vi "Targeting Unit.vi"(0 "Main Interface":T6, 1 "Focus and Tracking":T3, 2 "Guided Approach":T4, 3 "Controls":T1, 4 "Start Coordinates [pix]":refnum<vi>, 5 "Manipulator Interface":T10, 7 "Target":T9, 9 "Tip":T8, 11 "Error In":errorcluster, 12 "System of Reference Interface":T7, 13 "Calibration":T5, 14 "State":refnum<vi>) -> (15 "Error Out":errorcluster)   [LabVIEW 2012, in "Targeting Unit.lvlib"]
uses:
  Targeting Unit.lvlib
  <vilib>/Analysis/Matrix/Datatypes/RealMatrix.ctl
  State.ctl
  <vilib>/Analysis/Matrix/NI_Matrix.lvlib
panel:
  out "Final Reference [um]":T2
  out "Initial Reference [um]":T2
  out "Exit":bool
  out "XmF":dbl format="%.2f"
  out "XmI":dbl format="%.2f"
  out "Final [pix]":cluster{"X":sgl, "Y":sgl}
  out "Initial [pix]":cluster{"X":sgl, "Y":sgl}
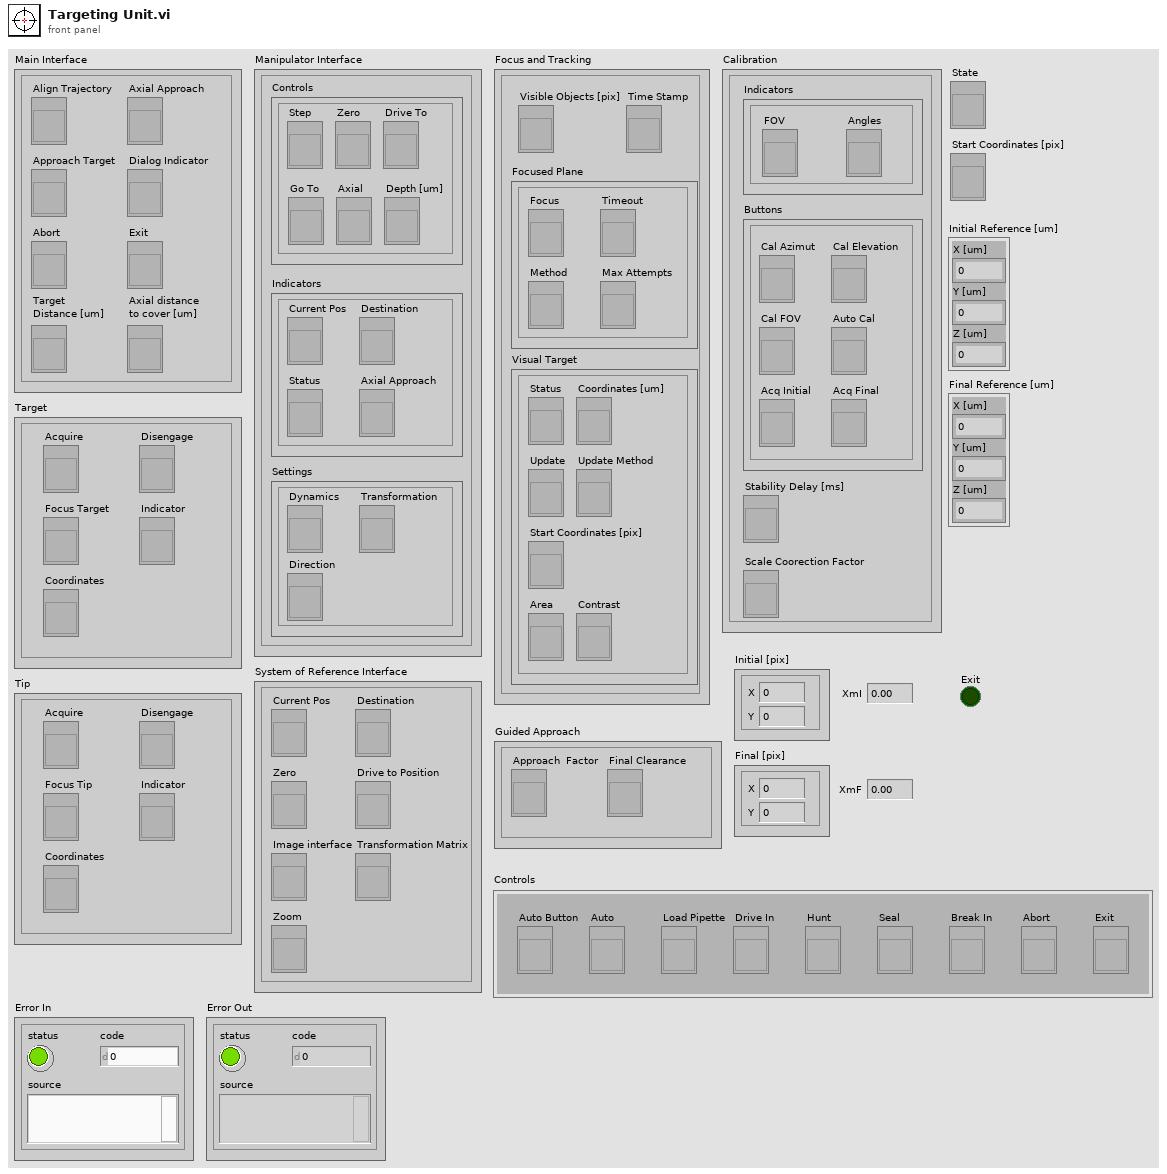
[diagram p1: front panel]
types:
  T1 = cluster{"Load Pipette":refnum<vi>, "Drive In":refnum<vi>, "Hunt":refnum<vi>, "Seal":refnum<vi>, "Break In":refnum<vi>, "Abort":refnum<vi>, "Exit":refnum<vi>, "Auto":refnum<vi>, "Auto Button":refnum<vi>}
  T2 = cluster{"X [um]":dbl, "Y [um]":dbl, "Z [um]":dbl}
  T3 = cluster{"Focused Plane":cluster{"Focus":refnum<vi>, "Timeout":refnum<vi>, "Max Attempts":refnum<vi>, "Method":refnum<vi>}, "Time Stamp":refnum<vi>, "Visual Target":cluster{"Coordinates [um]":refnum<vi>, "Status":refnum<vi>, "Update":refnum<vi>, "Update Method":refnum<vi>, "Start Coordinates [pix]":refnum<vi>, "Area":refnum<vi>, "Contrast":refnum<vi>}, "Visible Objects [pix]":refnum<vi>}
  T4 = cluster{"Approach  Factor":refnum<vi>, "Final Clearance":refnum<vi>}
  T5 = cluster{"Indicators":cluster{"FOV":refnum<vi>, "Angles":refnum<vi>}, "Buttons":cluster{"Cal FOV":refnum<vi>, "Cal Azimut":refnum<vi>, "Cal Elevation":refnum<vi>, "Auto Cal":refnum<vi>, "Acq Initial":refnum<vi>, "Acq Final":refnum<vi>}, "Stability Delay [ms]":refnum<vi>, "Scale Coorection Factor":refnum<vi>}
  T6 = cluster{"Exit":refnum<vi>, "Abort":refnum<vi>, "Align Trajectory":refnum<vi>, "Axial Approach":refnum<vi>, "Dialog Indicator":refnum<vi>, "Approach Target":refnum<vi>, "Target\nDistance [um]":refnum<vi>, "Axial distance\nto cover [um]":refnum<vi>}
  T7 = cluster{"Current Pos":refnum<vi>, "Image interface":refnum<vi>, "Transformation Matrix":refnum<vi>, "Zero":refnum<vi>, "Destination":refnum<vi>, "Drive to Position":refnum<vi>, "Zoom":refnum<vi>}
  T8 = cluster{"Coordinates":refnum<vi>, "Acquire":refnum<vi>, "Disengage":refnum<vi>, "Indicator":refnum<vi>, "Focus Tip":refnum<vi>}
  T9 = cluster{"Coordinates":refnum<vi>, "Acquire":refnum<vi>, "Disengage":refnum<vi>, "Indicator":refnum<vi>, "Focus Target":refnum<vi>}
  T10 = cluster{"Indicators":cluster{"Current Pos":refnum<vi>, "Destination":refnum<vi>, "Status":refnum<vi>, "Axial Approach":refnum<vi>}, "Settings":cluster{"Dynamics":refnum<vi>, "Transformation":refnum<vi>, "Direction":refnum<vi>}, "Controls":cluster{"Zero":refnum<vi>, "Step":refnum<vi>, "Drive To":refnum<vi>, "Go To":refnum<vi>, "Axial":refnum<vi>, "Depth [um]":refnum<vi>}}
  T11 = typedef "NI_Matrix.lvlib/RealMatrix.ctl" = dbl[][]
  T12 = cluster{"X [um]":bool, "Y [um]":bool, "Z [um]":bool}
  T13 = cluster{"Global Rectangle":i32[], "Contours":cluster{"Contour Type":u32, "ROI Type":u32, "Points":i32[]}[]}
  T14 = typedef "IMAQ Point" = cluster{"X":sgl, "Y":sgl}
  T15 = typedef "State.ctl" = enum16{"READY", "LOAD", "LOCALIZATION", "HUNTING", "SEAL", "BREAKIN", "WCR", "ALIGN", "APPROACH", "TARGETING"}
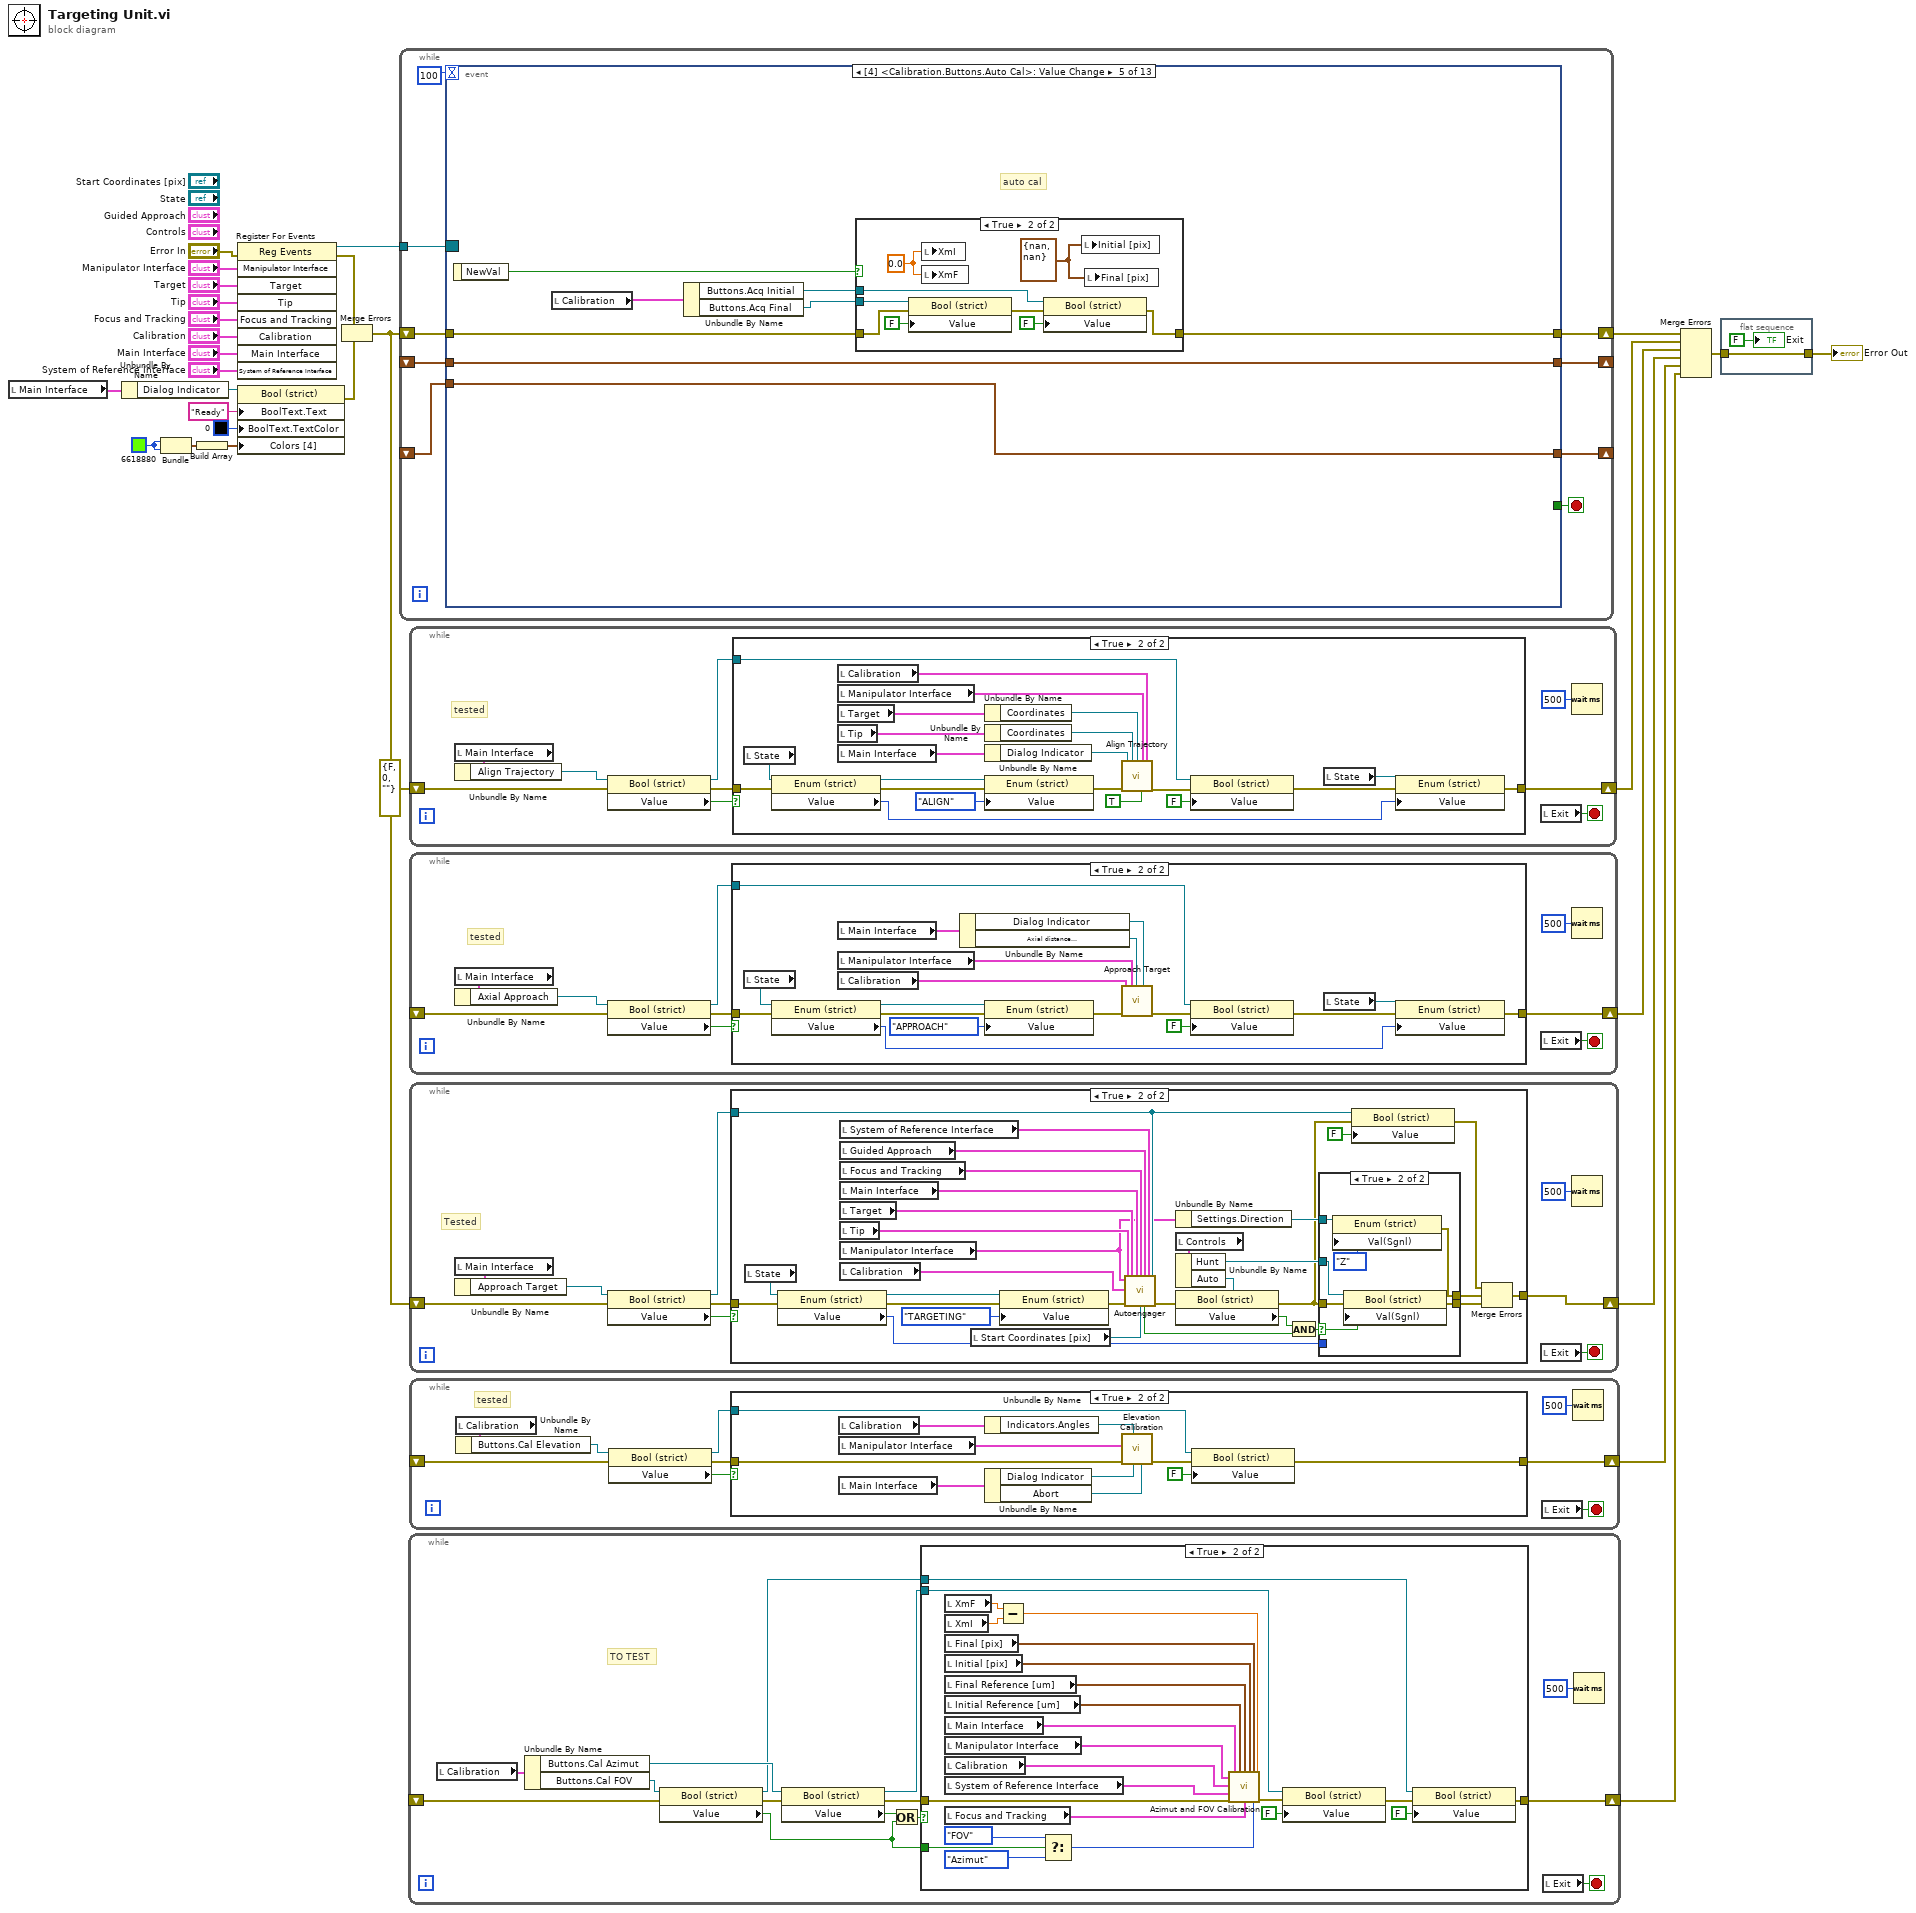
[diagram p0: block diagram]
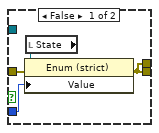
[diagram p3: hidden frame]
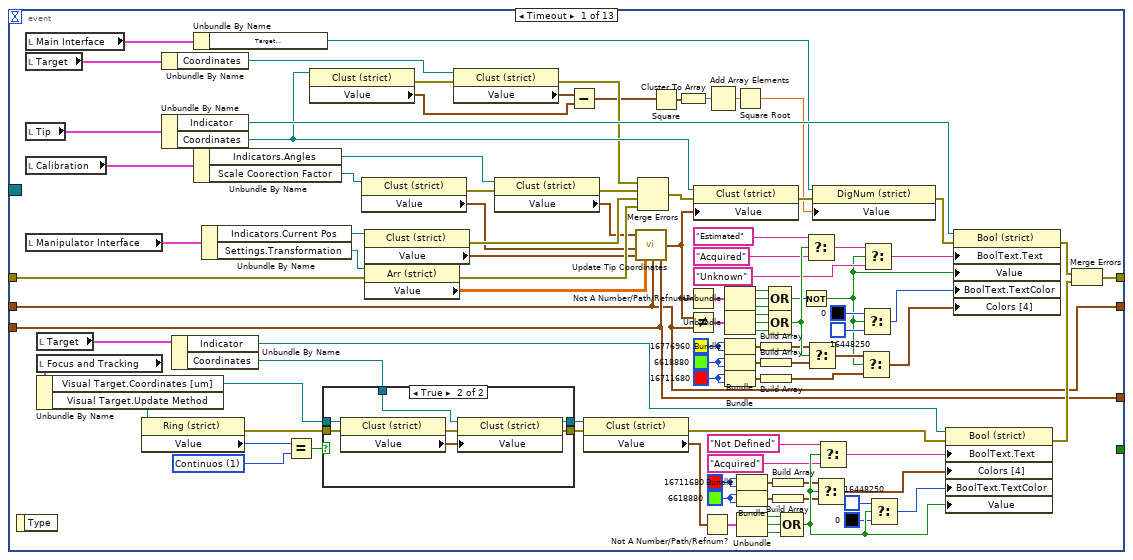
[diagram p8: hidden frame]
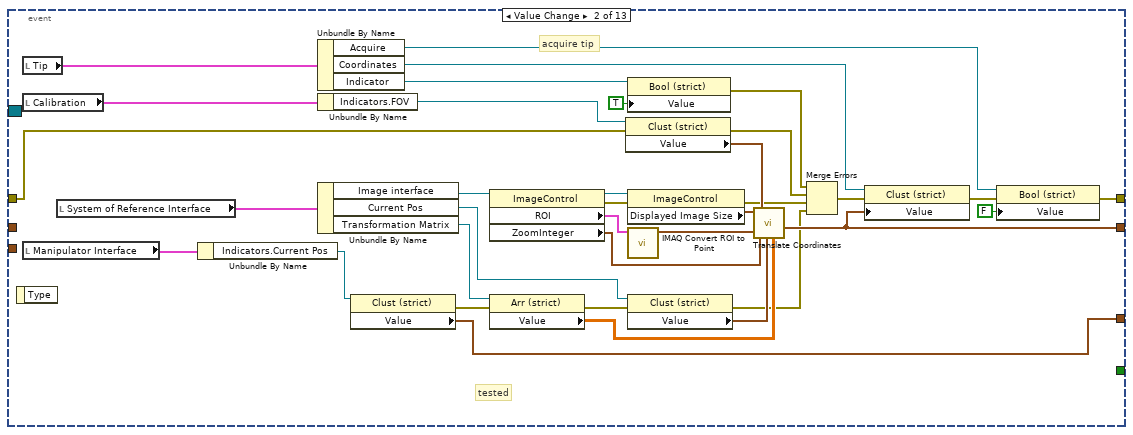
[diagram p10: hidden frame]
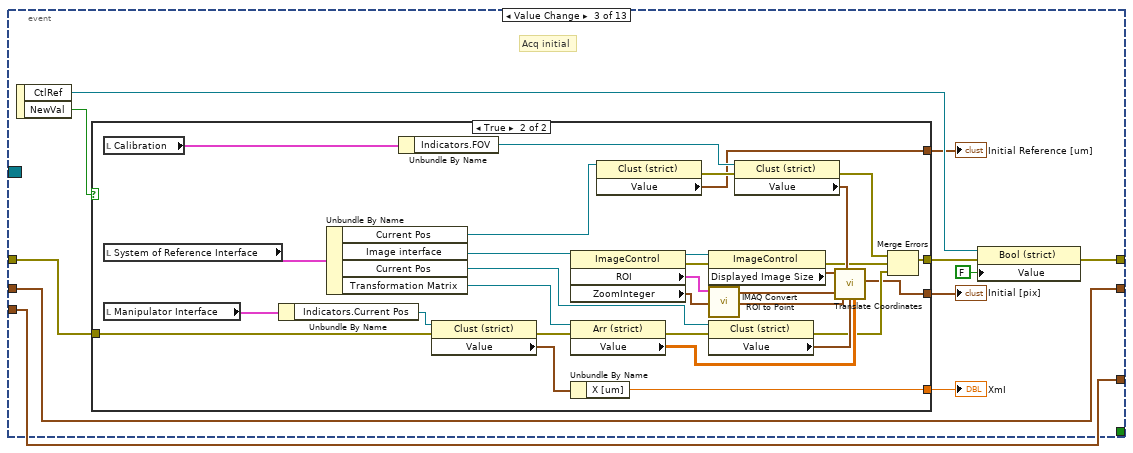
[diagram p11: hidden frame]
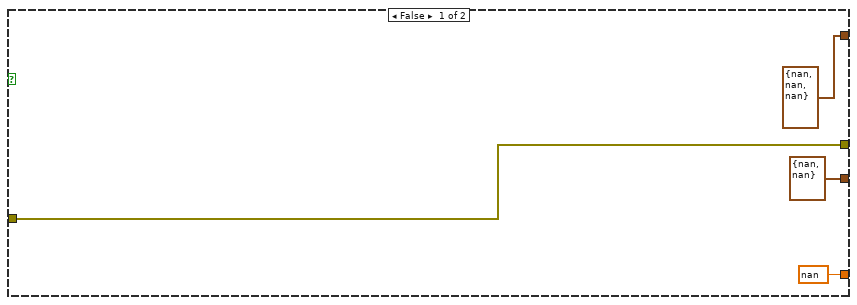
[diagram p12: hidden frame]
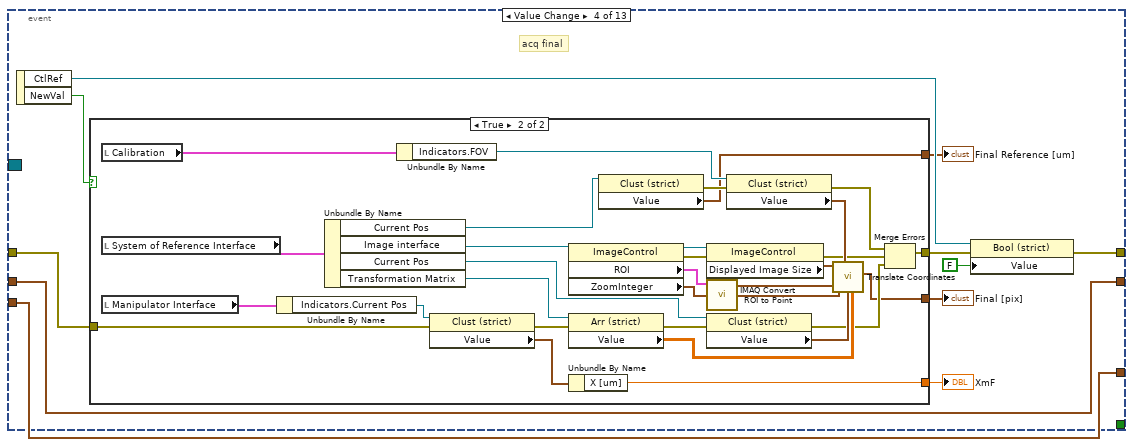
[diagram p13: hidden frame]
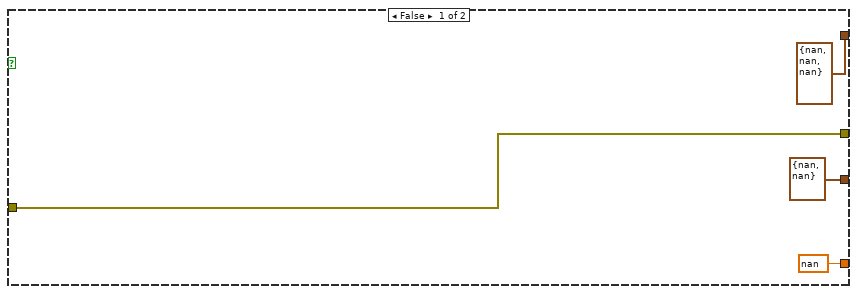
[diagram p14: hidden frame]
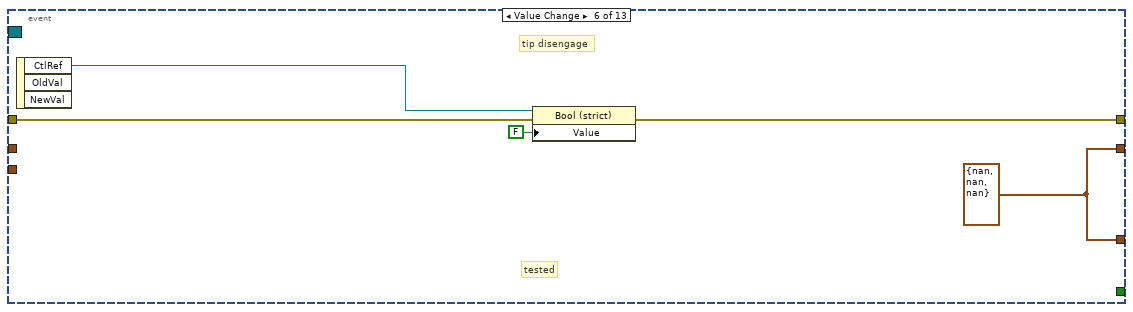
[diagram p16: hidden frame]
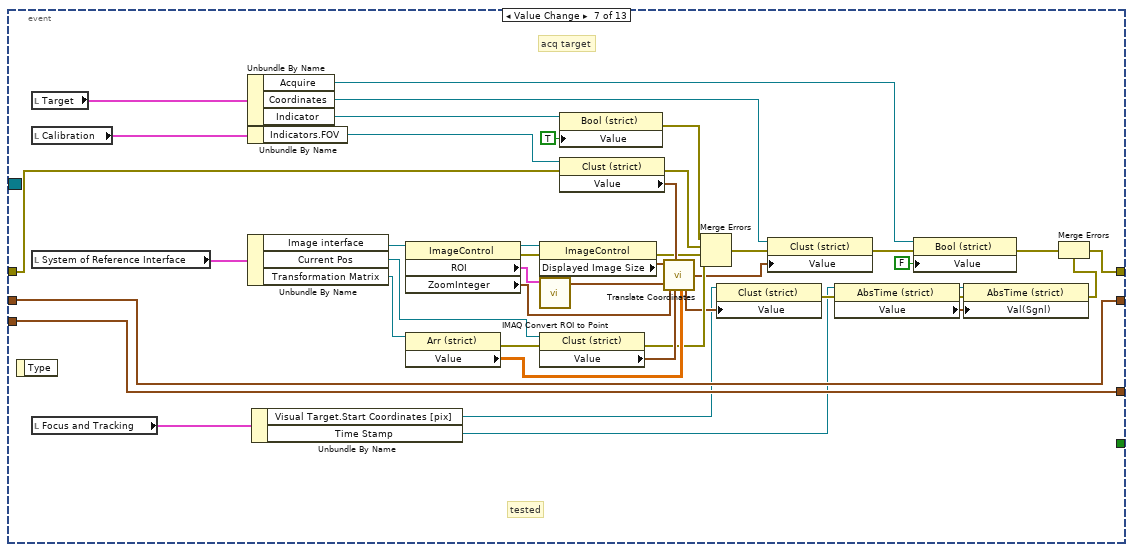
[diagram p17: hidden frame]
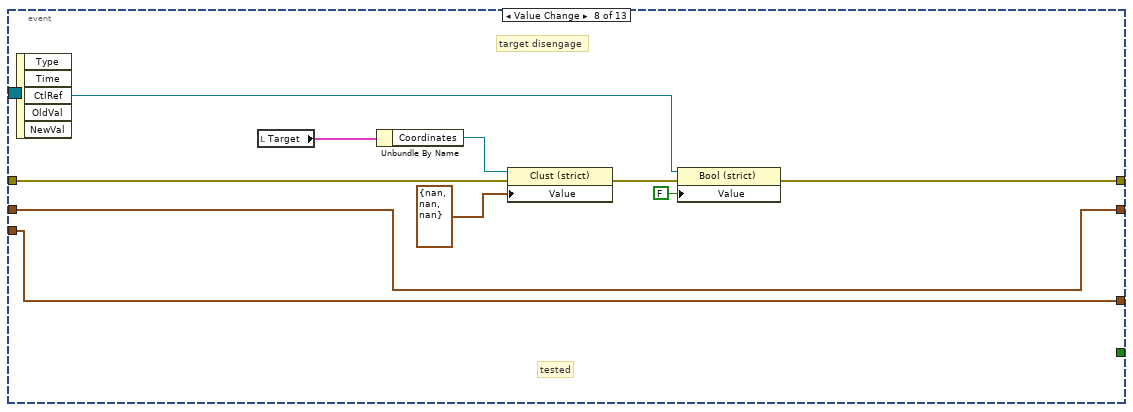
[diagram p18: hidden frame]
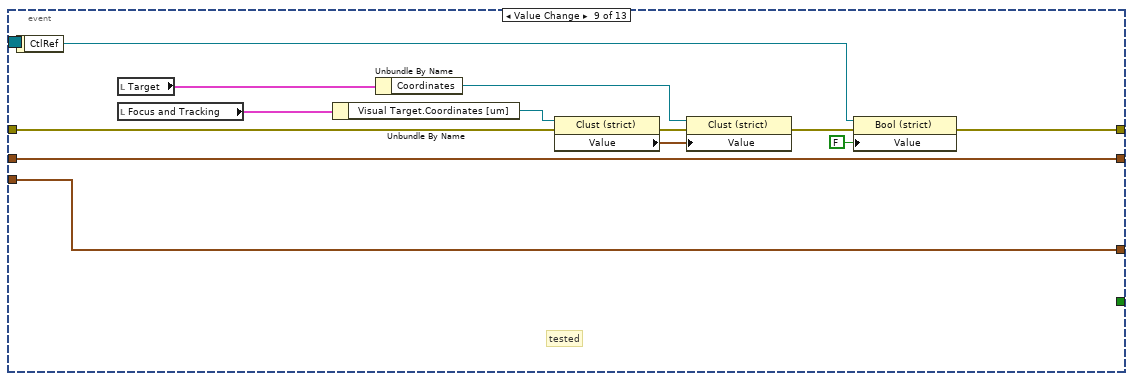
[diagram p19: hidden frame]
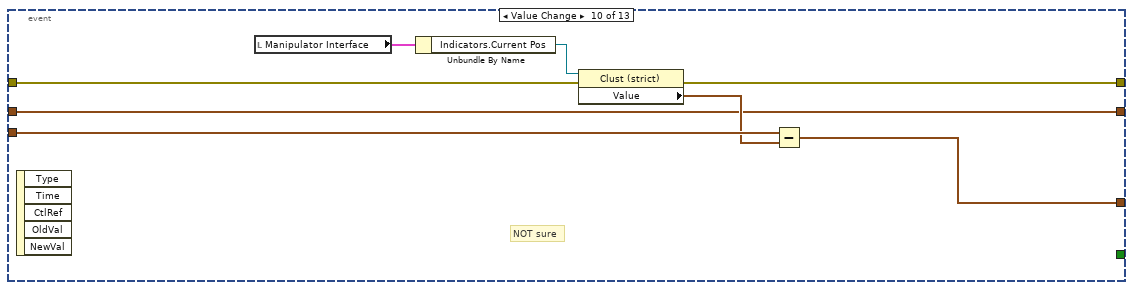
[diagram p20: hidden frame]
diagram:
  w8 = u32 6618880
  n1 = local read "Main Interface"() -> (w3:T6)
  n2 = Unbundle By Name(w3) -> ("Dialog Indicator"=w2:refnum<vi>)
  n3 = Bundle(w8, w8) -> (w7:cluster{u32, u32})  [unwired: 1 in]
  n4 = Build Array(w7) -> (w4:cluster{u32, u32}[])
  n5 = register-events(error in="Error In", "Manipulator Interface", "Target", "Tip", "Focus and Tracking", "Calibration", "Main Interface", "System of Reference Interface") -> (reference out=w23:refnum<event-registration>, error out=w18:errorcluster)  [unwired: 1 in]
  n6 = property class="Bool (strict)"(reference=w2, "BoolText.Text"="Ready" ("Boolean Text.Text"), "BoolText.TextColor"=u32 0, "Colors [4]"=w4) -> (error out=w6:errorcluster)  [unwired: 1 in, 1 out]
  n7 = Merge Errors(w18, w6) -> (w10:errorcluster)
  n8 = while {
    tunnel: w23 -> [w37]
    shift-right: [w35] -> _
    shift-left: _ -> [w34]
    shift-right: [w36] -> _
    shift-left: _ -> [w33]
    shift-right: [w32] -> w17
    shift-left: w10 -> [w29]
    stop <- w30 stop-if-true
    n9 = event shown="[4] <Calibration.Buttons.Auto Cal>: Value Change" {
      selector: w37 -> [_ _ _ _ _ _ _ _ _ _ _ _ _]
      dyn-events: _ -> [_ _ _ _ _ _ _ _ _ _ _ _ _]
      timeout: 100 -> [_ _ _ _ _ _ _ _ _ _ _ _ _]
      tunnel: [w57 w176 w186 w239 w280 w296 w313 w341 w355 w363 w374 w405 w422] -> w36
      tunnel: [w59 w150 w185 w237 w279 w296 w312 w342 w354 w370 w372 w404 w423] -> w35
      tunnel: w34 -> [w59 _ w185 w237 w279 _ w312 w342 w354 w369 w372 w404 w423]
      tunnel: w33 -> [w57 _ w186 w239 w280 _ w313 w341 w355 w363 w373 w405 w422]
      tunnel: [w73 w158 w190 w233 w276 w293 w301 w348 w352 w365 w379 w391 w425] -> w32
      tunnel: w29 -> [w87 w149 w192 w238 w277 w294 w297 w345 w356 w366 w383 w398 w425]
      tunnel: [_ _ _ _ _ _ _ _ _ _ _ _ w424] -> w30
      event Timeout {
        w63 = 1 items=["On Demand", "Continuos"] ("Target Update Method")
        w120 = u32 16711680
        w110 = u32 6618880
        w107 = u32 16776960
        w95 = u32 6618880
        w92 = u32 16711680
        n10 = event-data() -> ()  [unwired: 1 in, 1 out]
        n11 = local read "Main Interface"() -> (w38:T6)
        n12 = local read "Target"() -> (w47:T9)
        n13 = local read "Tip"() -> (w134:T8)
        n14 = local read "Calibration"() -> (w135:T5)
        n15 = local read "Manipulator Interface"() -> (w137:T10)
        n16 = local read "Target"() -> (w80:T9)
        n17 = local read "Focus and Tracking"() -> (w65:T3)
        n18 = Unbundle By Name(w65) -> ("Visual Target.Coordinates [um]"=w58:refnum<vi>, "Visual Target.Update Method"=w64:refnum<vi>)
        n19 = property class="Ring (strict)"(reference=w64) -> (error out=w61:errorcluster, "Value"=w62:i32)  [unwired: 1 in, 1 out]
        n20 = Unbundle By Name(w47) -> ("Coordinates"=w46:refnum<vi>)
        n21 = Unbundle By Name(w134) -> ("Indicator"=w72:refnum<vi>, "Coordinates"=w50:refnum<vi>)
        n22 = Unbundle By Name(w80) -> ("Indicator"=w69:refnum<vi>, "Coordinates"=w67:refnum<vi>)
        n23 = Unbundle By Name(w38) -> ("Target\nDistance [um]"=w44:refnum<vi>)
        n24 = Unbundle By Name(w135) -> ("Indicators.Angles"=w136:refnum<vi>, "Scale Coorection Factor"=w55:refnum<vi>)
        n25 = Unbundle By Name(w137) -> ("Indicators.Current Pos"=w139:refnum<vi>, "Settings.Transformation"=w138:refnum<vi>)
        n26 = Equal?(x=w62, y=w63) -> (x = y?=w60:bool)
        n27 = property class="Clust (strict)"(reference=w50) -> (error out=w45:errorcluster, "Value"=w42:T2)  [unwired: 1 in, 1 out]
        n28 = case shown="True" w60 {
          tunnel: [w141 w148] -> w68
          tunnel: w67 -> [w140 w146]
          tunnel: [w140 w147] -> w66
          tunnel: w58 -> [_ w145]
          tunnel: w61 -> [w141 w144]
          frame False {
          }
          frame True {
            n29 = property class="Clust (strict)"(reference=w145, error in=w144) -> (error out=w142:errorcluster, "Value"=w143:cluster{"X":dbl, "Y":dbl, "Z":dbl})  [unwired: 1 out]
            n30 = property class="Clust (strict)"(reference=w146, error in=w142, "Value"=w143) -> (reference out=w147:refnum<vi>, error out=w148:errorcluster)
          }
        }
        n31 = property class="Clust (strict)"(reference=w55) -> (error out=w56:errorcluster, "Value"=w54:cluster{"Kx":dbl, "Ky":dbl, "Kz":dbl})  [unwired: 1 in, 1 out]
        n32 = property class="Clust (strict)"(reference=w139) -> (error out=w85:errorcluster, "Value"=w82:T2)  [unwired: 1 in, 1 out]
        n33 = property class="Arr (strict)"(reference=w138, error in=w87) -> (error out=w84:errorcluster, "Value"=w133:T11)  [unwired: 1 out]
        n34 = property class="Clust (strict)"(reference=w46, error in=w45) -> (error out=w41:errorcluster, "Value"=w43:T2)  [unwired: 1 out]
        n35 = property class="Clust (strict)"(reference=w136, error in=w56) -> (error out=w86:errorcluster, "Value"=w83:cluster{"Azimut":dbl, "Elevation":dbl})  [unwired: 1 out]
        n36 = Subtract(x=w43, y=w42) -> (x-y=w40:T2)
        n37 = property class="Clust (strict)"(reference=w66, error in=w68) -> (error out=w70:errorcluster, "Value"=w101:T2)  [unwired: 1 out]
        n38 = call "Update Tip Coordinates.vi"("Scale Coorection Factor"=w54, "Angles"=w83, "Transformation Matrix"=w133, "Initial Manipulator Coordinates"=w59, "Initial Tip Coordinates"=w57, "Current Manipulator Coordinates"=w82) -> ("Current Coordinates"=w79:T2)  [unwired: 5 in]
        n39 = Merge Errors(w41, w86, w85, w84) -> (w81:errorcluster)
        n40 = Square(x=w40) -> (x^2=w51:T2)
        n41 = Cluster To Array(cluster=w51) -> (array=w52:dbl[])
        n42 = Not A Number/Path/Refnum?(number/path/refnum=w79) -> (NaN/Path/Refnum?=w115:T12)
        n43 = Not Equal?(x=w79, y=w57) -> (x != y?=w88:T12)
        n44 = property class="Clust (strict)"(reference=w50, error in=w81, "Value"=w79) -> (error out=w49:errorcluster)  [unwired: 1 out]
        n45 = Not A Number/Path/Refnum?(number/path/refnum=w101) -> (NaN/Path/Refnum?=w102:T12)
        n46 = Add Array Elements(numeric array=w52) -> (sum=w53:dbl)
        n47 = Unbundle(w115) -> ("X [um]"=w116:bool, "Y [um]"=w117:bool, "Z [um]"=w118:bool)
        n48 = Unbundle(w88) -> ("X [um]"=w89:bool, "Y [um]"=w90:bool, "Z [um]"=w91:bool)
        n49 = Bundle(w107, w107) -> (w108:cluster{u32, u32})  [unwired: 1 in]
        n50 = Bundle(w110, w110) -> (w111:cluster{u32, u32})  [unwired: 1 in]
        n51 = Bundle(w120, w120) -> (w121:cluster{u32, u32})  [unwired: 1 in]
        n52 = Square Root(x=w53) -> (sqrt(x)=w39:dbl)
        n53 = Bundle(w92, w92) -> (w93:cluster{u32, u32})  [unwired: 1 in]
        n54 = Bundle(w95, w95) -> (w96:cluster{u32, u32})  [unwired: 1 in]
        n55 = Unbundle(w102) -> ("X [um]"=w103:bool, "Y [um]"=w104:bool, "Z [um]"=w105:bool)
        n56 = Build Array(w108) -> (w109:cluster{u32, u32}[])
        n57 = Build Array(w111) -> (w112:cluster{u32, u32}[])
        n58 = Build Array(w121) -> (w124:cluster{u32, u32}[])
        n59 = Compound Arithmetic op=OR(w116, w117, w118) -> (w119:bool)
        n60 = Compound Arithmetic op=OR(w89, w90, w91) -> (w126:bool)
        n61 = Build Array(w93) -> (w94:cluster{u32, u32}[])
        n62 = Build Array(w96) -> (w97:cluster{u32, u32}[])
        n63 = Compound Arithmetic op=OR(w103, w104, w105) -> (w132:bool)
        n64 = Not(x=w119) -> (.not. x?=w77:bool)
        n65 = Select(t="Estimated" ("Boolean Text.Text"), s=w126, f="Acquired" ("Boolean Text.Text")) -> (s? t:f=w122:string)
        n66 = Select(t=w109, s=w126, f=w112) -> (s? t:f=w125:cluster{u32, u32}[])
        n67 = property class="DigNum (strict)"(reference=w44, error in=w49, "Value"=w39) -> (error out=w48:errorcluster)  [unwired: 1 out]
        n68 = Select(t=w94, s=w132, f=w97) -> (s? t:f=w100:cluster{u32, u32}[])
        n69 = Select(t="Not Defined" ("Boolean Text.Text"), s=w132, f="Acquired" ("Boolean Text.Text")) -> (s? t:f=w106:string)
        n70 = Select(t=w125, s=w77, f=w124) -> (s? t:f=w75:cluster{u32, u32}[])
        n71 = Select(t=u32 0, s=w77, f=u32 16448250) -> (s? t:f=w76:u32)
        n72 = Select(t=w122, s=w77, f="Unknown" ("Boolean Text.Text")) -> (s? t:f=w78:string)
        n73 = Select(t=u32 16448250, s=w132, f=u32 0) -> (s? t:f=w131:u32)
        n74 = property class="Bool (strict)"(reference=w69, error in=w70, "BoolText.Text"=w106, "Colors [4]"=w100, "BoolText.TextColor"=w131, "Value"=w132) -> (error out=w71:errorcluster)  [unwired: 1 out]
        n75 = property class="Bool (strict)"(reference=w72, error in=w48, "BoolText.Text"=w78, "Value"=w77, "BoolText.TextColor"=w76, "Colors [4]"=w75) -> (error out=w74:errorcluster)  [unwired: 1 out]
        n76 = Merge Errors(w74, w71) -> (w73:errorcluster)
      }
      event Value Change {
        # "acquire tip"
        # "tested"
        n77 = event-data() -> ()  [unwired: 1 in, 1 out]
        n78 = local read "Tip"() -> (w177:T8)
        n79 = local read "Calibration"() -> (w179:T5)
        n80 = local read "Manipulator Interface"() -> (w175:T10)
        n81 = local read "System of Reference Interface"() -> (w163:T7)
        n82 = Unbundle By Name(w175) -> ("Indicators.Current Pos"=w174:refnum<vi>)
        n83 = Unbundle By Name(w177) -> ("Acquire"=w173:refnum<vi>, "Coordinates"=w154:refnum<vi>, "Indicator"=w153:refnum<vi>)
        n84 = Unbundle By Name(w179) -> ("Indicators.FOV"=w178:refnum<vi>)
        n85 = Unbundle By Name(w163) -> ("Image interface"=w167:refnum<vi>, "Current Pos"=w157:refnum<vi>, "Transformation Matrix"=w172:refnum<vi>)
        n86 = property class="Clust (strict)"(reference=w174) -> (error out=w156:errorcluster, "Value"=w150:T2)  [unwired: 1 in, 1 out]
        n87 = property on="Property Node" class="ImageControl"(reference=w167) -> (reference out=w168:refnum<vi>, error out=w166:errorcluster, "ROI"=w180:T13, "ZoomInteger"=w151:cluster{"X":i32, "Y":i32})  [unwired: 1 in]
        n88 = property class="Arr (strict)"(reference=w172, error in=w156) -> (error out=w164:errorcluster, "Value"=w182:T11)  [unwired: 1 out]
        n89 = property class="Clust (strict)"(reference=w178, error in=w149) -> (error out=w162:errorcluster, "Value"=w171:cluster{"FOVx [um]":dbl, "FOVy [um]":dbl})  [unwired: 1 out]
        n90 = property class="Bool (strict)"(reference=w153, "Value"=TRUE) -> (error out=w152:errorcluster)  [unwired: 1 in, 1 out]
        n91 = property class="ImageControl"(reference=w168, error in=w166) -> (error out=w161:errorcluster, "Displayed Image Size"=w169:cluster{"Width":u32, "Height":u32})  [unwired: 1 out]
        n92 = call "IMAQ Convert ROI to Point"("ROI Descriptor"=w180) -> ("Point"=w170:T14)  [unwired: 1 in, 8 out]
        n93 = property class="Clust (strict)"(reference=w157, error in=w164) -> (error out=w159:errorcluster, "Value"=w165:T2)  [unwired: 1 out]
        n94 = call "Translate Coordinates.vi"("Transformation Matrix"=w182, "Coordinates [pix]"=w170, "FOV"=w171, "Visualiser Zoom"=w151, "Scope Position"=w165, "Image Area"=w169) -> ("Target Coordinates"=w176:T2)  [unwired: 4 in, 1 out]
        n95 = Merge Errors(w152, w162, w161, w159) -> (w160:errorcluster)
        n96 = property class="Clust (strict)"(reference=w154, error in=w160, "Value"=w176) -> (error out=w155:errorcluster)  [unwired: 1 out]
        n97 = property class="Bool (strict)"(reference=w173, error in=w155, "Value"=FALSE) -> (error out=w158:errorcluster)  [unwired: 1 out]
      }
      event Value Change {
        # "Acq initial"
        n98 = event-data() -> ("CtlRef"=w188:refnum<vi>, "NewVal"=w191:bool)  [unwired: 1 in]
        n99 = case shown="True" w191 {
          tunnel: [w198 w207] -> w189
          tunnel: [cluster{"X":sgl, "Y":sgl} {"X"=nan, "Y"=nan} ("coordinates [pix]") w203] -> w194
          tunnel: [nan ("X [um]") w205] -> w193
          tunnel: w192 -> [w198 w204]
          tunnel: [T2 {"X [um]"=nan, "Y [um]"=nan, "Z [um]"=nan} ("Value") w200] -> w184
          frame False {
          }
          frame True {
            n100 = local read "Calibration"() -> (w226:T5)
            n101 = local read "System of Reference Interface"() -> (w213:T7)
            n102 = local read "Manipulator Interface"() -> (w224:T10)
            n103 = Unbundle By Name(w224) -> ("Indicators.Current Pos"=w223:refnum<vi>)
            n104 = Unbundle By Name(w213) -> ("Current Pos"=w202:refnum<vi>, "Image interface"=w217:refnum<vi>, "Current Pos"=w209:refnum<vi>, "Transformation Matrix"=w222:refnum<vi>)
            n105 = Unbundle By Name(w226) -> ("Indicators.FOV"=w225:refnum<vi>)
            n106 = property class="Clust (strict)"(reference=w223, error in=w204) -> (error out=w208:errorcluster, "Value"=w206:T2)  [unwired: 1 out]
            n107 = property on="Property Node" class="ImageControl"(reference=w217) -> (reference out=w218:refnum<vi>, error out=w216:errorcluster, "ROI"=w227:T13, "ZoomInteger"=w199:cluster{"X":i32, "Y":i32})  [unwired: 1 in]
            n108 = property class="Arr (strict)"(reference=w222, error in=w208) -> (error out=w214:errorcluster, "Value"=w228:T11)  [unwired: 1 out]
            n109 = Unbundle By Name(w206) -> ("X [um]"=w205:dbl)
            n110 = property class="Clust (strict)"(reference=w202) -> (error out=w201:errorcluster, "Value"=w200:T2)  [unwired: 1 in, 1 out]
            n111 = property class="ImageControl"(reference=w218, error in=w216) -> (error out=w211:errorcluster, "Displayed Image Size"=w219:cluster{"Width":u32, "Height":u32})  [unwired: 1 out]
            n112 = call "IMAQ Convert ROI to Point"("ROI Descriptor"=w227) -> ("Point"=w220:T14)  [unwired: 1 in, 8 out]
            n113 = property class="Clust (strict)"(reference=w209, error in=w214) -> (error out=w210:errorcluster, "Value"=w215:T2)  [unwired: 1 out]
            n114 = property class="Clust (strict)"(reference=w225, error in=w201) -> (error out=w212:errorcluster, "Value"=w221:cluster{"FOVx [um]":dbl, "FOVy [um]":dbl})  [unwired: 1 out]
            n115 = call "Translate Coordinates.vi"("Transformation Matrix"=w228, "Coordinates [pix]"=w220, "FOV"=w221, "Visualiser Zoom"=w199, "Scope Position"=w215, "Image Area"=w219) -> ("coordinates [pix]"=w203:cluster{"X":sgl, "Y":sgl})  [unwired: 4 in, 1 out]
            n116 = Merge Errors(w212, w211, w210) -> (w207:errorcluster)
          }
        }
        "Initial [pix]" <- w194
        "XmI" <- w193
        "Initial Reference [um]" <- w184
        n117 = property class="Bool (strict)"(reference=w188, error in=w189, "Value"=FALSE) -> (error out=w190:errorcluster)  [unwired: 1 out]
      }
      event Value Change {
        # "acq final"
        n118 = event-data() -> ("CtlRef"=w230:refnum<vi>, "NewVal"=w231:bool)  [unwired: 1 in]
        n119 = case shown="True" w231 {
          tunnel: [w243 w252] -> w232
          tunnel: [cluster{"X":sgl, "Y":sgl} {"X"=nan, "Y"=nan} ("coordinates [pix]") w251] -> w236
          tunnel: [nan ("X [um]") w249] -> w235
          tunnel: w238 -> [w243 w248]
          tunnel: [T2 {"X [um]"=nan, "Y [um]"=nan, "Z [um]"=nan} ("Value") w245] -> w229
          frame False {
          }
          frame True {
            n120 = local read "Calibration"() -> (w271:T5)
            n121 = local read "System of Reference Interface"() -> (w258:T7)
            n122 = local read "Manipulator Interface"() -> (w269:T10)
            n123 = Unbundle By Name(w269) -> ("Indicators.Current Pos"=w268:refnum<vi>)
            n124 = Unbundle By Name(w258) -> ("Current Pos"=w246:refnum<vi>, "Image interface"=w262:refnum<vi>, "Current Pos"=w254:refnum<vi>, "Transformation Matrix"=w267:refnum<vi>)
            n125 = Unbundle By Name(w271) -> ("Indicators.FOV"=w270:refnum<vi>)
            n126 = property class="Clust (strict)"(reference=w268, error in=w248) -> (error out=w253:errorcluster, "Value"=w250:T2)  [unwired: 1 out]
            n127 = property on="Property Node" class="ImageControl"(reference=w262) -> (reference out=w263:refnum<vi>, error out=w261:errorcluster, "ROI"=w272:T13, "ZoomInteger"=w244:cluster{"X":i32, "Y":i32})  [unwired: 1 in]
            n128 = property class="Arr (strict)"(reference=w267, error in=w253) -> (error out=w259:errorcluster, "Value"=w273:T11)  [unwired: 1 out]
            n129 = Unbundle By Name(w250) -> ("X [um]"=w249:dbl)
            n130 = property class="Clust (strict)"(reference=w246) -> (error out=w247:errorcluster, "Value"=w245:T2)  [unwired: 1 in, 1 out]
            n131 = property class="ImageControl"(reference=w263, error in=w261) -> (error out=w256:errorcluster, "Displayed Image Size"=w264:cluster{"Width":u32, "Height":u32})  [unwired: 1 out]
            n132 = call "IMAQ Convert ROI to Point"("ROI Descriptor"=w272) -> ("Point"=w265:T14)  [unwired: 1 in, 8 out]
            n133 = property class="Clust (strict)"(reference=w254, error in=w259) -> (error out=w255:errorcluster, "Value"=w260:T2)  [unwired: 1 out]
            n134 = property class="Clust (strict)"(reference=w270, error in=w247) -> (error out=w257:errorcluster, "Value"=w266:cluster{"FOVx [um]":dbl, "FOVy [um]":dbl})  [unwired: 1 out]
            n135 = call "Translate Coordinates.vi"("Transformation Matrix"=w273, "Coordinates [pix]"=w265, "FOV"=w266, "Visualiser Zoom"=w244, "Scope Position"=w260, "Image Area"=w264) -> ("coordinates [pix]"=w251:cluster{"X":sgl, "Y":sgl})  [unwired: 4 in, 1 out]
            n136 = Merge Errors(w257, w256, w255) -> (w252:errorcluster)
          }
        }
        "Final [pix]" <- w236
        "XmF" <- w235
        "Final Reference [um]" <- w229
        n137 = property class="Bool (strict)"(reference=w230, error in=w232, "Value"=FALSE) -> (error out=w233:errorcluster)  [unwired: 1 out]
      }
      event Value Change {
        # "auto cal"
        n138 = event-data() -> ("NewVal"=w281:bool)  [unwired: 1 in]
        n139 = local read "Calibration"() -> (w278:T5)
        n140 = Unbundle By Name(w278) -> ("Buttons.Acq Initial"=w274:refnum<vi>, "Buttons.Acq Final"=w275:refnum<vi>)
        n141 = case shown="True" w281 {
          tunnel: w277 -> [w282 w289]
          tunnel: [w282 w287] -> w276
          tunnel: w275 -> [_ w286]
          tunnel: w274 -> [_ w285]
          frame False {
          }
          frame True {
            w290 = 0.0 ("XmI")
            w291 = cluster{"X":sgl, "Y":sgl} {"X"=nan, "Y"=nan} ("Initial [pix]")
            n142 = property class="Bool (strict)"(reference=w286, error in=w289, "Value"=FALSE) -> (error out=w288:errorcluster)  [unwired: 1 out]
            n143 = local write "XmI"(w290) -> ()
            n144 = local write "XmF"(w290) -> ()
            n145 = property class="Bool (strict)"(reference=w285, error in=w288, "Value"=FALSE) -> (error out=w287:errorcluster)  [unwired: 1 out]
            n146 = local write "Initial [pix]"(w291) -> ()
            n147 = local write "Final [pix]"(w291) -> ()
          }
        }
      }
      event Value Change {
        w296 = T2 {"X [um]"=nan, "Y [um]"=nan, "Z [um]"=nan} ("Value")
        # "tip disengage"
        # "tested"
        n148 = event-data() -> ("CtlRef"=w292:refnum<vi>)  [unwired: 1 in, 2 out]
        n149 = property class="Bool (strict)"(reference=w292, error in=w294, "Value"=FALSE) -> (error out=w293:errorcluster)  [unwired: 1 out]
      }
      event Value Change {
        # "acq target"
        # "tested"
        n150 = event-data() -> ()  [unwired: 1 in, 1 out]
        n151 = local read "Target"() -> (w333:T9)
        n152 = local read "Calibration"() -> (w335:T5)
        n153 = local read "System of Reference Interface"() -> (w322:T7)
        n154 = local read "Focus and Tracking"() -> (w311:T3)
        n155 = Unbundle By Name(w333) -> ("Acquire"=w332:refnum<vi>, "Coordinates"=w316:refnum<vi>, "Indicator"=w315:refnum<vi>)
        n156 = Unbundle By Name(w335) -> ("Indicators.FOV"=w334:refnum<vi>)
        n157 = Unbundle By Name(w322) -> ("Image interface"=w326:refnum<vi>, "Current Pos"=w317:refnum<vi>, "Transformation Matrix"=w331:refnum<vi>)
        n158 = Unbundle By Name(w311) -> ("Visual Target.Start Coordinates [pix]"=w308:refnum<vi>, "Time Stamp"=w303:refnum<vi>)
        n159 = property on="Property Node" class="ImageControl"(reference=w326) -> (reference out=w327:refnum<vi>, error out=w325:errorcluster, "ROI"=w336:T13, "ZoomInteger"=w298:cluster{"X":i32, "Y":i32})  [unwired: 1 in]
        n160 = property class="Arr (strict)"(reference=w331) -> (error out=w323:errorcluster, "Value"=w338:T11)  [unwired: 1 in, 1 out]
        n161 = property class="ImageControl"(reference=w327, error in=w325) -> (error out=w320:errorcluster, "Displayed Image Size"=w328:cluster{"Width":u32, "Height":u32})  [unwired: 1 out]
        n162 = call "IMAQ Convert ROI to Point"("ROI Descriptor"=w336) -> ("Point"=w329:T14)  [unwired: 1 in, 8 out]
        n163 = property class="Clust (strict)"(reference=w317, error in=w323) -> (error out=w318:errorcluster, "Value"=w324:T2)  [unwired: 1 out]
        n164 = property class="Bool (strict)"(reference=w315, "Value"=TRUE) -> (error out=w314:errorcluster)  [unwired: 1 in, 1 out]
        n165 = property class="Clust (strict)"(reference=w334, error in=w297) -> (error out=w321:errorcluster, "Value"=w330:cluster{"FOVx [um]":dbl, "FOVy [um]":dbl})  [unwired: 1 out]
        n166 = call "Translate Coordinates.vi"("Transformation Matrix"=w338, "Coordinates [pix]"=w329, "FOV"=w330, "Visualiser Zoom"=w298, "Scope Position"=w324, "Image Area"=w328) -> ("Target Coordinates"=w309:T2, "coordinates [pix]"=w310:cluster{"X":sgl, "Y":sgl})  [unwired: 4 in]
        n167 = Merge Errors(w314, w321, w320, w318) -> (w319:errorcluster)
        n168 = property class="Clust (strict)"(reference=w308, "Value"=w310) -> (error out=w304:errorcluster)  [unwired: 1 in, 1 out]
        n169 = property class="Clust (strict)"(reference=w316, error in=w319, "Value"=w309) -> (error out=w302:errorcluster)  [unwired: 1 out]
        n170 = property class="AbsTime (strict)"(reference=w303, error in=w304) -> (reference out=w307:refnum<vi>, error out=w306:errorcluster, "Value"=w305:timestamp)
        n171 = property class="Bool (strict)"(reference=w332, error in=w302, "Value"=FALSE) -> (error out=w300:errorcluster)  [unwired: 1 out]
        n172 = property class="AbsTime (strict)"(reference=w307, error in=w306, "Val(Sgnl)"=w305) -> (error out=w299:errorcluster)  [unwired: 1 out]
        n173 = Merge Errors(w300, w299) -> (w301:errorcluster)
      }
      event Value Change {
        # "target disengage"
        # "tested"
        n174 = event-data() -> ("CtlRef"=w340:refnum<vi>)  [unwired: 1 in, 4 out]
        n175 = local read "Target"() -> (w344:T9)
        n176 = Unbundle By Name(w344) -> ("Coordinates"=w343:refnum<vi>)
        n177 = property class="Clust (strict)"(reference=w343, error in=w345, "Value"=T2 {"X [um]"=nan, "Y [um]"=nan, "Z [um]"=nan}) -> (error out=w346:errorcluster)  [unwired: 1 out]
        n178 = property class="Bool (strict)"(reference=w340, error in=w346, "Value"=FALSE) -> (error out=w348:errorcluster)  [unwired: 1 out]
      }
      event Value Change {
        # "tested"
        n179 = event-data() -> ("CtlRef"=w351:refnum<vi>)  [unwired: 1 in]
        n180 = local read "Target"() -> (w362:T9)
        n181 = local read "Focus and Tracking"() -> (w360:T3)
        n182 = Unbundle By Name(w360) -> ("Visual Target.Coordinates [um]"=w359:refnum<vi>)
        n183 = Unbundle By Name(w362) -> ("Coordinates"=w361:refnum<vi>)
        n184 = property class="Clust (strict)"(reference=w359, error in=w356) -> (error out=w357:errorcluster, "Value"=w358:cluster{"X":dbl, "Y":dbl, "Z":dbl})  [unwired: 1 out]
        n185 = property class="Clust (strict)"(reference=w361, error in=w357, "Value"=w358) -> (error out=w353:errorcluster)  [unwired: 1 out]
        n186 = property class="Bool (strict)"(reference=w351, error in=w353, "Value"=FALSE) -> (error out=w352:errorcluster)  [unwired: 1 out]
      }
      event Value Change {
        # "NOT sure"
        n187 = event-data() -> ()  [unwired: 1 in, 5 out]
        n188 = local read "Manipulator Interface"() -> (w367:T10)
        n189 = Unbundle By Name(w367) -> ("Indicators.Current Pos"=w368:refnum<vi>)
        n190 = property class="Clust (strict)"(reference=w368, error in=w366) -> (error out=w365:errorcluster, "Value"=w364:T2)  [unwired: 1 out]
        n191 = Subtract(x=w369, y=w364) -> (x-y=w370:T2)
      }
      event Value Change {
        # "initial manip"
        # "initial tip"
        # "Tested"
        n192 = event-data() -> ()  [unwired: 1 in, 5 out]
        n193 = local read "Target"() -> (w381:T9)
        n194 = local read "System of Reference Interface"() -> (w384:T7)
        n195 = Unbundle By Name(w381) -> ("Coordinates"=w378:refnum<vi>)
        n196 = Unbundle By Name(w384) -> ("Current Pos"=w385:refnum<vi>)
        n197 = property class="Clust (strict)"(reference=w385, error in=w383) -> (error out=w380:errorcluster, "Value"=w371:T2)  [unwired: 1 out]
        n198 = property class="Clust (strict)"(reference=w378, error in=w380) -> (reference out=w377:refnum<vi>, error out=w382:errorcluster, "Value"=w376:T2)
        n199 = Subtract(x=w376, y=w371) -> (x-y=w375:T2)
        n200 = Subtract(x=w373, y=w371) -> (x-y=w374:T2)
        n201 = property class="Clust (strict)"(reference=w377, error in=w382, "Value"=w375) -> (error out=w379:errorcluster)  [unwired: 1 out]
      }
      event Value Change {
        n202 = event-data() -> ()  [unwired: 1 in, 5 out]
        n203 = local read "Focus and Tracking"() -> (w390:T3)
        n204 = local read "System of Reference Interface"() -> (w389:T7)
        n205 = flat-sequence {
          tunnel: [w421] -> w399
          tunnel: w398 -> [w421]
          frame #0 {
            n206 = Wait (ms)(milliseconds to wait=u32 500) -> ()  [unwired: 1 out]
          }
        }
        n207 = Unbundle By Name(w390) -> ("Visual Target.Start Coordinates [pix]"=w394:refnum<vi>)
        n208 = Unbundle By Name(w389) -> ("Image interface"=w406:refnum<vi>)
        n209 = property on="Property Node" class="ImageControl"(reference=w406, error in=w399) -> (error out=w407:errorcluster, "Displayed Image Size"=w402:cluster{"Width":u32, "Height":u32}, "ZoomInteger"=w401:cluster{"X":i32, "Y":i32})  [unwired: 1 out]
        n210 = Divide(x=w402, y=w401) -> (x/y=w400:cluster{dbl, dbl})
        n211 = Divide(x=w400, y=2.0) -> (x/y=w397:cluster{dbl, dbl})
        n212 = property class="Clust (strict)"(reference=w394, error in=w407, "Value"=w397) -> (error out=w396:errorcluster)  [unwired: 1 out]
        n213 = flat-sequence {
          tunnel: [w419] -> w395
          tunnel: w396 -> [w419]
          frame #0 {
            n214 = Wait (ms)(milliseconds to wait=u32 3000) -> ()  [unwired: 1 out]
          }
        }
        n215 = property class="Clust (strict)"(reference=w394, error in=w395, "Value"=w397) -> (error out=w393:errorcluster)  [unwired: 1 out]
        n216 = local read "Start Coordinates [pix]"() -> (w387:refnum<vi>)
        n217 = local read "Calibration"() -> (w388:T5)
        n218 = local read "Target"() -> (w386:T9)
        n219 = flat-sequence {
          tunnel: [w417] -> w392
          tunnel: w393 -> [w417]
          frame #0 {
            n220 = Wait (ms)(milliseconds to wait=u32 3000) -> ()  [unwired: 1 out]
          }
        }
        n221 = disable-structure shown="Disabled" {
          disable-tunnel: w392 -> [w414 w415]
          disable-tunnel: [w413 w415] -> w391
          disable-tunnel: w390 -> [w412 _]
          disable-tunnel: w389 -> [w411 _]
          disable-tunnel: w388 -> [w410 _]
          disable-tunnel: w387 -> [w409 _]
          disable-tunnel: w386 -> [w408 _]
          frame Disabled {
            n222 = call "Place Target On Nearest Visible Object.vi"("Focus and Tracking"=w412, "Start Coordinates [pix]"=w409, "System of Reference Interface"=w411, "Calibration"=w410, "Target"=w408, "error in (no error)"=w414) -> ("error out"=w413:errorcluster)  [unwired: 8 in, 1 out]
          }
          frame Enabled {
          }
        }
      }
      event Value Change {
        w424 = TRUE ("NewVal")
        n223 = event-data() -> ()  [unwired: 1 in, 5 out]
        n224 = local write "Exit"(w424) -> ()
      }
    }
  }
  n225 = while {
    shift-right: [w434] -> w16
    shift-left: _ -> [w429]
    stop <- w438 stop-if-true
    # "TO TEST"
    n226 = local read "Calibration"() -> (w435:T5)
    n227 = Unbundle By Name(w435) -> ("Buttons.Cal Azimut"=w436:refnum<vi>, "Buttons.Cal FOV"=w428:refnum<vi>)
    n228 = property class="Bool (strict)"(reference=w428, error in=w429) -> (reference out=w427:refnum<vi>, error out=w430:errorcluster, "Value"=w426:bool)
    n229 = property class="Bool (strict)"(reference=w436, error in=w430) -> (reference out=w433:refnum<vi>, error out=w437:errorcluster, "Value"=w432:bool)
    n230 = Or(x=w432, y=w426) -> (x .or. y?=w431:bool)
    n231 = case shown="True" w431 {
      tunnel: [w440 w452] -> w434
      tunnel: w437 -> [w440 w442]
      tunnel: w433 -> [_ w455]
      tunnel: w427 -> [_ w451]
      tunnel: w426 -> [_ w448]
      frame False {
      }
      frame True {
        n232 = local read "XmF"() -> (w458:dbl)
        n233 = local read "XmI"() -> (w459:dbl)
        n234 = local read "Final [pix]"() -> (w460:cluster{"X":sgl, "Y":sgl})
        n235 = local read "Initial [pix]"() -> (w461:cluster{"X":sgl, "Y":sgl})
        n236 = local read "Final Reference [um]"() -> (w443:T2)
        n237 = local read "Initial Reference [um]"() -> (w444:T2)
        n238 = local read "Main Interface"() -> (w463:T6)
        n239 = local read "Manipulator Interface"() -> (w464:T10)
        n240 = local read "Calibration"() -> (w462:T5)
        n241 = local read "System of Reference Interface"() -> (w441:T7)
        n242 = local read "Focus and Tracking"() -> (w445:T3)
        n243 = Subtract(x=w458, y=w459) -> (x-y=w446:dbl)
        n244 = Select(t=enum16{"Azimut", "FOV", "Azimut and FOV"}."FOV" ("Parameters"), s=w448, f=enum16{"Azimut", "FOV", "Azimut and FOV"}."Azimut" ("Parameters")) -> (s? t:f=w447:enum16{"Azimut", "FOV", "Azimut and FOV"})
        n245 = call "Azimut and FOV Calibration.vi"("Main Interface"=w463, "Manipulator Interface"=w464, "Calibration"=w462, "Parameters"=w447, "Focus and Tracking"=w445, "Error In"=w442, "Distance [um]"=w446, "System of Reference Interface"=w441, "Initial [pix]"=w461, "Final [pix]"=w460, "Initial Reference [um]"=w444, "Final Reference [um]"=w443) -> ("Error Out"=w456:errorcluster)  [unwired: 7 in]
        n246 = property class="Bool (strict)"(reference=w455, error in=w456, "Value"=FALSE) -> (error out=w453:errorcluster)  [unwired: 1 out]
        n247 = property class="Bool (strict)"(reference=w451, error in=w453, "Value"=FALSE) -> (error out=w452:errorcluster)  [unwired: 1 out]
      }
    }
    n248 = local read "Exit"() -> (w438:bool)
    n249 = Wait (ms)(milliseconds to wait=u32 500) -> ()  [unwired: 1 out]
  }
  n250 = while {
    shift-right: [w466] -> w12
    shift-left: errorcluster {"status"=FALSE, "code"=0, "source"=""} ("error out") -> [w469]
    stop <- w468 stop-if-true
    # "tested"
    n251 = local read "Main Interface"() -> (w473:T6)
    n252 = Unbundle By Name(w473) -> ("Align Trajectory"=w472:refnum<vi>)
    n253 = property class="Bool (strict)"(reference=w472, error in=w469) -> (reference out=w465:refnum<vi>, error out=w470:errorcluster, "Value"=w471:bool)
    n254 = case shown="True" w471 {
      tunnel: w470 -> [w474 w479]
      tunnel: [w474 w484] -> w466
      tunnel: w465 -> [_ w487]
      frame False {
      }
      frame True {
        n255 = local read "State"() -> (w478:refnum<vi>)
        n256 = property class="Enum (strict)"(reference=w478, error in=w479) -> (reference out=w480:refnum<vi>, error out=w481:errorcluster, "Value"=w477:T15)
        n257 = local read "Calibration"() -> (w486:T5)
        n258 = local read "Manipulator Interface"() -> (w496:T10)
        n259 = local read "Target"() -> (w493:T9)
        n260 = local read "Tip"() -> (w492:T8)
        n261 = local read "Main Interface"() -> (w490:T6)
        n262 = Unbundle By Name(w493) -> ("Coordinates"=w494:refnum<vi>)
        n263 = Unbundle By Name(w492) -> ("Coordinates"=w495:refnum<vi>)
        n264 = Unbundle By Name(w490) -> ("Dialog Indicator"=w491:refnum<vi>)
        n265 = property class="Enum (strict)"(reference=w480, error in=w481, "Value"=State."ALIGN") -> (error out=w485:errorcluster)  [unwired: 1 out]
        n266 = call "Align Trajectory.vi"("Force alignemnt"=TRUE, "Indicator"=w491, "Calibration"=w486, "error in"=w485, "Tip Coordinates"=w495, "Target Coordinates"=w494, "Manipulator Interface"=w496) -> ("error out"=w488:errorcluster)  [unwired: 3 in, 1 out]
        n267 = property class="Bool (strict)"(reference=w487, error in=w488, "Value"=FALSE) -> (error out=w483:errorcluster)  [unwired: 1 out]
        n268 = local read "State"() -> (w482:refnum<vi>)
        n269 = property class="Enum (strict)"(reference=w482, error in=w483, "Value"=w477) -> (error out=w484:errorcluster)  [unwired: 1 out]
      }
    }
    n270 = local read "Exit"() -> (w468:bool)
    n271 = Wait (ms)(milliseconds to wait=u32 500) -> ()  [unwired: 1 out]
  }
  n272 = while {
    shift-right: [w498] -> w13
    shift-left: _ -> [w501]
    stop <- w500 stop-if-true
    # "tested"
    n273 = local read "Main Interface"() -> (w505:T6)
    n274 = Unbundle By Name(w505) -> ("Axial Approach"=w504:refnum<vi>)
    n275 = property class="Bool (strict)"(reference=w504, error in=w501) -> (reference out=w497:refnum<vi>, error out=w502:errorcluster, "Value"=w503:bool)
    n276 = case shown="True" w503 {
      tunnel: w502 -> [w506 w512]
      tunnel: [w506 w509] -> w498
      tunnel: w497 -> [_ w520]
      frame False {
      }
      frame True {
        n277 = local read "State"() -> (w513:refnum<vi>)
        n278 = property class="Enum (strict)"(reference=w513, error in=w512) -> (reference out=w516:refnum<vi>, error out=w515:errorcluster, "Value"=w508:T15)
        n279 = local read "Main Interface"() -> (w523:T6)
        n280 = local read "Manipulator Interface"() -> (w524:T10)
        n281 = local read "Calibration"() -> (w519:T5)
        n282 = Unbundle By Name(w523) -> ("Dialog Indicator"=w518:refnum<vi>, "Axial distance\nto cover [um]"=w517:refnum<vi>)
        n283 = property class="Enum (strict)"(reference=w516, error in=w515, "Value"=State."APPROACH") -> (error out=w514:errorcluster)  [unwired: 1 out]
        n284 = call "Approach Target.vi"("Indicator"=w518, "Axial distance [um]"=w517, "error in"=w514, "Calibration"=w519, "Manipulator Interface"=w524) -> ("error out"=w521:errorcluster)  [unwired: 5 in, 1 out]
        n285 = property class="Bool (strict)"(reference=w520, error in=w521, "Value"=FALSE) -> (error out=w510:errorcluster)  [unwired: 1 out]
        n286 = local read "State"() -> (w511:refnum<vi>)
        n287 = property class="Enum (strict)"(reference=w511, error in=w510, "Value"=w508) -> (error out=w509:errorcluster)  [unwired: 1 out]
      }
    }
    n288 = local read "Exit"() -> (w500:bool)
    n289 = Wait (ms)(milliseconds to wait=u32 500) -> ()  [unwired: 1 out]
  }
  n290 = while {
    shift-right: [w528] -> w14
    shift-left: w10 -> [w530]
    stop <- w532 stop-if-true
    # "Tested"
    n291 = local read "Main Interface"() -> (w529:T6)
    n292 = Unbundle By Name(w529) -> ("Approach Target"=w526:refnum<vi>)
    n293 = property class="Bool (strict)"(reference=w526, error in=w530) -> (reference out=w527:refnum<vi>, error out=w531:errorcluster, "Value"=w525:bool)
    n294 = case shown="True" w525 {
      tunnel: [w534 w544] -> w528
      tunnel: w531 -> [w534 w555]
      tunnel: w527 -> [_ w559]
      frame False {
      }
      frame True {
        n295 = local read "State"() -> (w552:refnum<vi>)
        n296 = property class="Enum (strict)"(reference=w552, error in=w555) -> (reference out=w553:refnum<vi>, error out=w554:errorcluster, "Value"=w546:T15)
        n297 = local read "System of Reference Interface"() -> (w558:T7)
        n298 = local read "Guided Approach"() -> (w562:T4)
        n299 = local read "Focus and Tracking"() -> (w560:T3)
        n300 = local read "Main Interface"() -> (w564:T6)
        n301 = local read "Target"() -> (w565:T9)
        n302 = local read "Tip"() -> (w557:T8)
        n303 = local read "Manipulator Interface"() -> (w540:T10)
        n304 = local read "Calibration"() -> (w563:T5)
        n305 = local read "Start Coordinates [pix]"() -> (w535:refnum<vi>)
        n306 = property class="Enum (strict)"(reference=w553, error in=w554, "Value"=State."TARGETING") -> (error out=w556:errorcluster)  [unwired: 1 out]
        n307 = call "Autoengager.vi"("Main Interface"=w564, "Focus and Tracking"=w560, "System of Reference Interface"=w558, "Guided Approach Calibration"=w562, "Approach Target Button"=w559, "Target"=w565, "Tip"=w557, "Error In"=w556, "Manipulator Interface"=w540, "Start Coordinates [pix]"=w535, "Calibration"=w563) -> ("Done"=w541:bool, "Error Out"=w547:errorcluster)  [unwired: 1 in, 2 out]
        n308 = Unbundle By Name(w540) -> ("Settings.Direction"=w539:refnum<vi>)
        n309 = local read "Controls"() -> (w550:T1)
        n310 = Unbundle By Name(w550) -> ("Hunt"=w548:refnum<vi>, "Auto"=w549:refnum<vi>)
        n311 = property class="Bool (strict)"(reference=w549, error in=w547) -> (error out=w536:errorcluster, "Value"=w543:bool)  [unwired: 1 out]
        n312 = And(x=w543, y=w541) -> (x .and. y?=w542:bool)
        n313 = case shown="True" w542 {
          selector: w542 -> [_ w574]
          tunnel: w536 -> [w569 w576]
          tunnel: w548 -> [_ w575]
          tunnel: [w566 w573] -> w545
          tunnel: w546 -> [w568 _]
          tunnel: w539 -> [_ w572]
          tunnel: [w566 w570] -> w537
          frame False {
            n314 = local read "State"() -> (w567:refnum<vi>)
            n315 = property class="Enum (strict)"(reference=w567, error in=w569, "Value"=w568) -> (error out=w566:errorcluster)  [unwired: 1 out]
          }
          frame True {
            n316 = property class="Enum (strict)"(reference=w572, "Val(Sgnl)"=enum16{"Z", "Axial"}."Z" ("Value (Signaling)")) -> (error out=w570:errorcluster)  [unwired: 1 in, 1 out]
            n317 = property class="Bool (strict)"(reference=w575, error in=w576, "Val(Sgnl)"=w574) -> (error out=w573:errorcluster)  [unwired: 1 out]
          }
        }
        n318 = property class="Bool (strict)"(reference=w559, error in=w536, "Value"=FALSE) -> (error out=w538:errorcluster)  [unwired: 1 out]
        n319 = Merge Errors(w538, w537, w545) -> (w544:errorcluster)
      }
    }
    n320 = local read "Exit"() -> (w532:bool)
    n321 = Wait (ms)(milliseconds to wait=u32 500) -> ()  [unwired: 1 out]
  }
  n322 = while {
    shift-right: [w578] -> w15
    shift-left: _ -> [w581]
    stop <- w585 stop-if-true
    # "tested"
    n323 = local read "Calibration"() -> (w583:T5)
    n324 = Unbundle By Name(w583) -> ("Buttons.Cal Elevation"=w584:refnum<vi>)
    n325 = property class="Bool (strict)"(reference=w584, error in=w581) -> (reference out=w577:refnum<vi>, error out=w582:errorcluster, "Value"=w580:bool)
    n326 = case shown="True" w580 {
      tunnel: [w586 w589] -> w578
      tunnel: w582 -> [w586 w592]
      tunnel: w577 -> [_ w587]
      frame False {
      }
      frame True {
        n327 = local read "Calibration"() -> (w597:T5)
        n328 = local read "Manipulator Interface"() -> (w595:T10)
        n329 = local read "Main Interface"() -> (w594:T6)
        n330 = Unbundle By Name(w597) -> ("Indicators.Angles"=w596:refnum<vi>)
        n331 = Unbundle By Name(w594) -> ("Dialog Indicator"=w591:refnum<vi>, "Abort"=w593:refnum<vi>)
        n332 = call "Elevation Calibration.vi"("Abort"=w593, "Dialog Indicator"=w591, "Angles"=w596, "error in"=w592, "Manipulator Interface"=w595) -> ("error out"=w590:errorcluster)  [unwired: 6 in]
        n333 = property class="Bool (strict)"(reference=w587, error in=w590, "Value"=FALSE) -> (error out=w589:errorcluster)  [unwired: 1 out]
      }
    }
    n334 = local read "Exit"() -> (w585:bool)
    n335 = Wait (ms)(milliseconds to wait=u32 500) -> ()  [unwired: 1 out]
  }
  n336 = Merge Errors(w17, w12, w13, w14, w15, w16) -> (w27:errorcluster)
  n337 = flat-sequence {
    tunnel: [w599] -> w28
    tunnel: w27 -> [w599]
    frame #0 {
      "Exit" <- FALSE ("Exit")
    }
  }
  "Error Out" <- w28
